vi "Triang Search_Check Input.vi"(0 "X In":dbl[](array[numeric]), 5 "Y In":dbl[](array[numeric]), 7 "Triangles In":i32[][](array[numeric]), 9 "Xi":dbl[](array[numeric]), 11 "Yi":dbl[](array[numeric])) -> (4 "X Out":dbl[](array[numeric]), 6 "Y Out":dbl[](array[numeric]), 8 "Triangles Out":i32[][](array[numeric]), 10 "Xi Out":dbl[](array[numeric]), 14 "error":i32, 15 "Yi Out":dbl[](array[numeric]))   [LabVIEW 2017, in "NI_AAL_Geometry.lvlib"]
uses:
  <vilib>/Analysis/NI_AAL_Geometry.lvlib
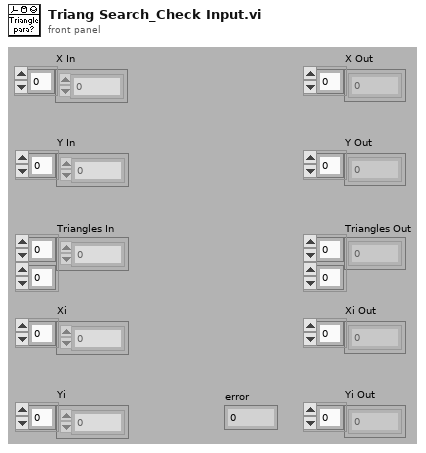
[diagram p1: front panel]
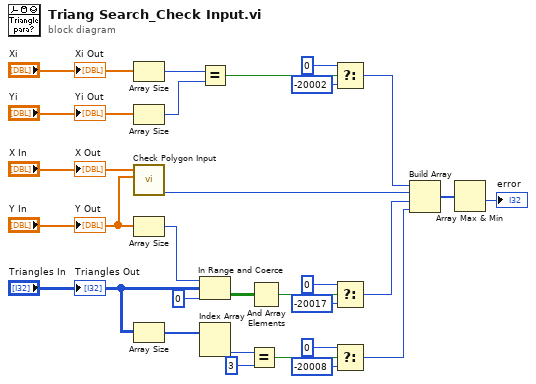
[diagram p0: block diagram]
diagram:
  n1 = Array Size(array="Xi") -> (size(s)=w28:i32)
  n2 = Array Size(array="Yi") -> (size(s)=w27:i32)
  n3 = call <vilib>:"Check Polygon Input.vi"("Y In"="Y In", "X In"="X In") -> ("error"=w5:i32)  [unwired: 7 in, 2 out]
  n4 = Array Size(array="Y In") -> (size(s)=w18:i32)
  n5 = Array Size(array="Triangles In") -> (size(s)=w13:i32[])
  n6 = Equal?(x=w28, y=w27) -> (x = y?=w17:bool)
  n7 = In Range and Coerce(upper limit=w18, x="Triangles In", lower limit=0) -> (In Range?=w23:bool[][])  [unwired: 1 out]
  n8 = Index Array(array=w13) -> (element #2=w12:i32)  [unwired: 2 in, 1 out]
  n9 = Equal?(x=w12, y=3) -> (x = y?=w9:bool)
  n10 = And Array Elements(Boolean array=w23) -> (logical AND=w21:bool)
  n11 = Select(t=0, s=w17, f=-20002) -> (s? t:f=w6:i32)
  n12 = Select(t=0, s=w21, f=-20017) -> (s? t:f=w4:i32)
  n13 = Select(t=0, s=w9, f=-20008) -> (s? t:f=w3:i32)
  n14 = Build Array(w6, w5, w4, w3) -> (w2:i32[])
  n15 = Array Max & Min(array=w2) -> (min value=→"error":i32)  [unwired: 3 out]
  "X Out" <- "X In"
  "Y Out" <- "Y In"
  "Triangles Out" <- "Triangles In"
  "Xi Out" <- "Xi"
  "Yi Out" <- "Yi"
